vi "SeCrTs-NS Write.vi"(8 "error in":errorcluster, 9 "to":enum16{"Storage", "Pumb", "Both"}(ring)=enum."Pumb", 10 "Data":variant, 11 "Message":string) -> (0 "error out":errorcluster)   [LabVIEW 2022 SP3]
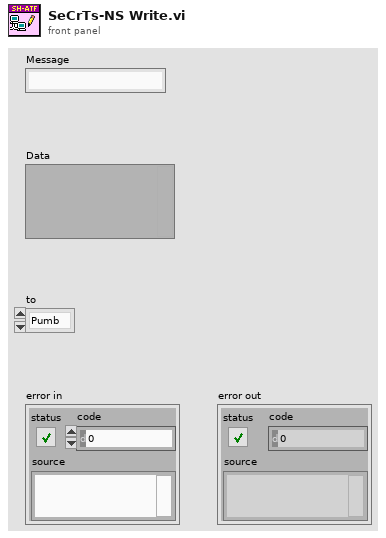
[diagram p1: front panel]
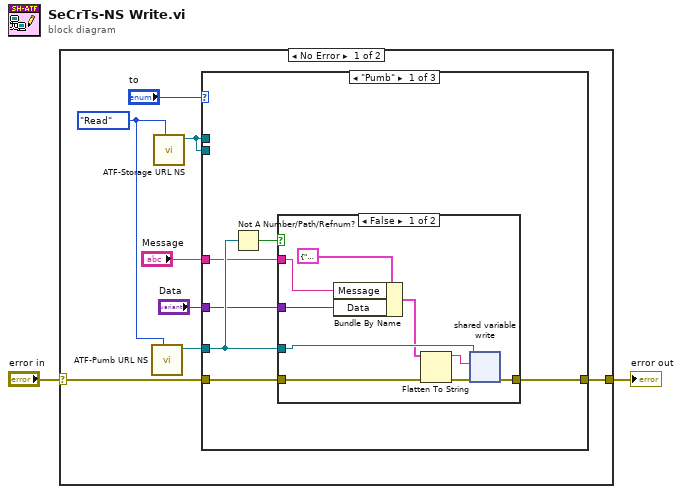
[diagram p0: block diagram]
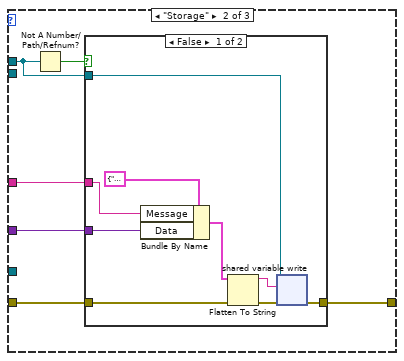
[diagram p3: hidden frame]
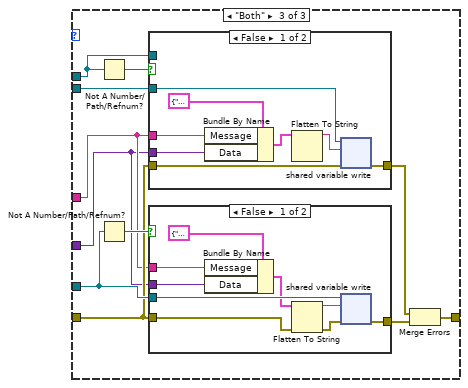
[diagram p5: hidden frame]
diagram:
  n1 = case shown="No Error" "error in" {
    selector: "error in" -> [w9 w73]
    tunnel: [w10 w73] -> w2
    frame No Error {
      w4 = enum16{"Init", "Read", "Write"}."Read" ("Enum")
      n2 = call "ATF-Pumb URL NS.vi"("Enum"=w4) -> ("writer endpoint 2"=w5:refnum<k21>)  [unwired: 9 in, 1 out]
      n3 = call "ATF-Storage URL NS.vi"("Enum"=w4) -> ("writer endpoint R"=w3:refnum<k21>)  [unwired: 9 in, 1 out]
      n4 = case shown="\"Pumb\"" "to" {
        tunnel: w5 -> [w15 _ w52]
        tunnel: w3 -> [_ w27 w50]
        tunnel: w9 -> [w14 w31 w49]
        tunnel: [w13 w30 w46] -> w10
        tunnel: "Message" -> [w12 w29 w45]
        tunnel: "Data" -> [w11 w28 w44]
        tunnel: w3 -> [_ _ w43]
        frame "Pumb" {
          n5 = Not A Number/Path/Refnum?(number/path/refnum=w15) -> (NaN/Path/Refnum?=w16:bool)
          n6 = case shown="False" w16 {
            tunnel: w15 -> [w25 _]
            tunnel: w14 -> [w20 w26]
            tunnel: [w23 w26] -> w13
            tunnel: w12 -> [w22 _]
            tunnel: w11 -> [w21 _]
            frame False {
              n7 = Bundle By Name(cluster=cluster{"Message":string, "Data":variant} {"Message"="", "Data"=variant}, "Message"=w22, "Data"=w21) -> (w17:cluster{"Message":string, "Data":variant})
              n8 = Flatten To String(anything=w17, error in (no error)=w20) -> (data string=w18:string, error out=w19:errorcluster)  [unwired: 2 in, 1 out]
              n9 = shared-variable-write(w25, w19, w18) -> (w23:errorcluster)  [unwired: 1 in, 2 out]
            }
            frame True {
            }
          }
        }
        frame "Storage" {
          n10 = Not A Number/Path/Refnum?(number/path/refnum=w27) -> (NaN/Path/Refnum?=w32:bool)
          n11 = case shown="False" w32 {
            tunnel: w27 -> [w41 _]
            tunnel: w31 -> [w35 w42]
            tunnel: [w39 w42] -> w30
            tunnel: w29 -> [w38 _]
            tunnel: w28 -> [w37 _]
            frame False {
              n12 = Bundle By Name(cluster=cluster{"Message":string, "Data":variant} {"Message"="", "Data"=variant}, "Message"=w38, "Data"=w37) -> (w33:cluster{"Message":string, "Data":variant})
              n13 = Flatten To String(anything=w33, error in (no error)=w35) -> (data string=w36:string, error out=w34:errorcluster)  [unwired: 2 in, 1 out]
              n14 = shared-variable-write(w41, w34, w36) -> (w39:errorcluster)  [unwired: 1 in, 2 out]
            }
            frame True {
            }
          }
        }
        frame "Both" {
          n15 = Not A Number/Path/Refnum?(number/path/refnum=w50) -> (NaN/Path/Refnum?=w51:bool)
          n16 = Not A Number/Path/Refnum?(number/path/refnum=w52) -> (NaN/Path/Refnum?=w53:bool)
          n17 = case shown="False" w51 {
            tunnel: w50 -> [_ _]
            tunnel: w49 -> [w56 w62]
            tunnel: [w55 w62] -> w48
            tunnel: w45 -> [w60 _]
            tunnel: w44 -> [w59 _]
            tunnel: w43 -> [w54 _]
            frame False {
              n18 = Bundle By Name(cluster=cluster{"Message":string, "Data":variant} {"Message"="", "Data"=variant}, "Message"=w60, "Data"=w59) -> (w58:cluster{"Message":string, "Data":variant})
              n19 = Flatten To String(anything=w58) -> (data string=w57:string)  [unwired: 3 in, 2 out]
              n20 = shared-variable-write(w54, w56, w57) -> (w55:errorcluster)  [unwired: 1 in, 2 out]
            }
            frame True {
            }
          }
          n21 = case shown="False" w53 {
            tunnel: w52 -> [w71 _]
            tunnel: w49 -> [w64 w72]
            tunnel: [w69 w72] -> w47
            tunnel: w45 -> [w67 _]
            tunnel: w44 -> [w68 _]
            frame False {
              n22 = Bundle By Name(cluster=cluster{"Message":string, "Data":variant} {"Message"="", "Data"=variant}, "Message"=w67, "Data"=w68) -> (w66:cluster{"Message":string, "Data":variant})
              n23 = Flatten To String(anything=w66, error in (no error)=w64) -> (data string=w65:string, error out=w63:errorcluster)  [unwired: 2 in, 1 out]
              n24 = shared-variable-write(w71, w63, w65) -> (w69:errorcluster)  [unwired: 1 in, 2 out]
            }
            frame True {
            }
          }
          n25 = Merge Errors(w48, w47) -> (w46:errorcluster)
        }
      }
    }
    frame Error {
    }
  }
  "error out" <- w2
